vi "Untitled 1.vi"() -> ()   [LabVIEW 2015]
panel:
  out "JSON string":string
  in  "REQUEST":T1
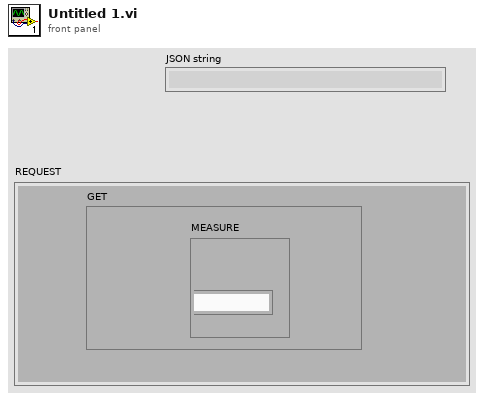
[diagram p1: front panel]
types:
  T1 = cluster{"GET":cluster{"MEASURE":cluster{"SN":string}}}
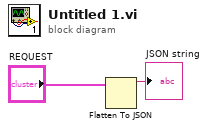
[diagram p0: block diagram]
diagram:
  n1 = Flatten To JSON(anything="REQUEST") -> (JSON string=→"JSON string":string)  [unwired: 2 in, 1 out]
